vi "Force2VoltageTrans.vi"(11 "force":dbl) -> (3 "voltage":dbl)   [LabVIEW 2019]
panel:
  # "This Vi calculates from a desired translational force the necessary voltage output for the motor."
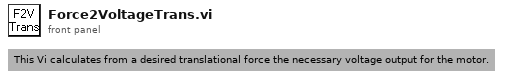
[diagram p1: front panel]
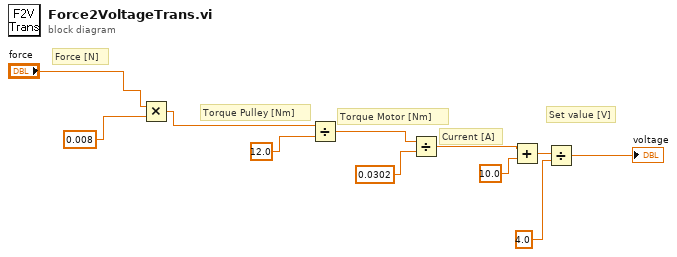
[diagram p0: block diagram]
diagram:
  # "Set value [V]"
  # "Torque Motor [Nm]"
  # "Torque Pulley [Nm]"
  # "Current [A]"
  # "Force [N]"
  n1 = Multiply(x="force", y=0.008) -> (x*y=w1:dbl)
  n2 = Divide(x=w1, y=12.0 ("value")) -> (x/y=w10:dbl)
  n3 = Divide(x=w10, y=0.0302) -> (x/y=w8:dbl)
  n4 = Add(x=w8, y=10.0) -> (x+y=w7:dbl)
  n5 = Divide(x=w7, y=4.0) -> (x/y=→"voltage":dbl)
